vi "Util Convert to Base64url No Padding.vi"(11 "String (hex display)":string) -> (3 "Base64url String":string)   [LabVIEW 2020, in "Netatmo-WeatherStation.lvlib"]
doc: "This VI converts a string to its Base64 equivalent. Base64 strings are commonly used in Internet protocols such as HTTP, SMTP, etc."
uses:
  Netatmo-WeatherStation.lvlib
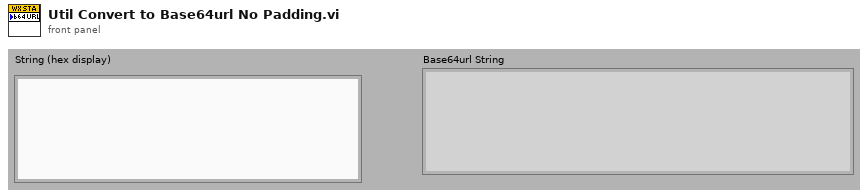
[diagram p1: front panel]
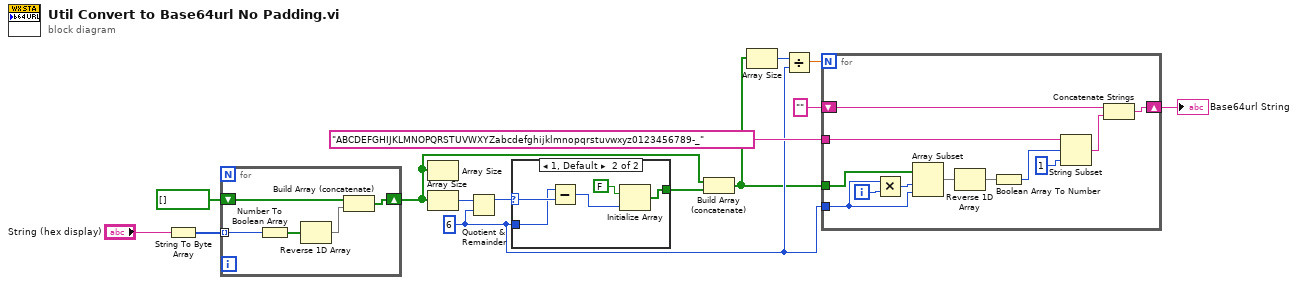
[diagram p0: block diagram]
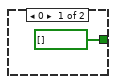
[diagram p2: hidden frame]
diagram:
  w4 = 6 ("y")
  n1 = String To Byte Array(string="String (hex display)") -> (unsigned byte array=w13:u8[])
  n2 = for {
    tunnel: w13 -> [w19] mode=indexing
    shift-right: [w16] -> w1
    shift-left: bool[] [] -> [w18]
    n3 = Number To Boolean Array(number=w19) -> (Boolean array=w17:bool[])
    n4 = Reverse 1D Array(array=w17) -> (reversed array=w15:bool[])
    n5 = Build Array (concatenate)(w18, w15) -> (w16:bool[])
  }
  n6 = Array Size(array=w1) -> ()  [unwired: 1 out]
  n7 = Array Size(array=w1) -> (size(s)=w7:i32)
  n8 = Quotient & Remainder(x=w7, y=w4) -> (x-y*floor(x/y)=w6:i32)  [unwired: 1 out]
  n9 = case shown="1, Default" w6 {
    selector: w6 -> [_ w24]
    tunnel: [bool[] [] w21] -> w5
    tunnel: w4 -> [_ w23]
    frame 0 {
    }
    frame 1, Default {
      n10 = Subtract(x=w23, y=w24) -> (x-y=w25:i32)
      n11 = Initialize Array(FALSE, w25) -> (w21:bool[])
    }
  }
  n12 = Build Array (concatenate)(w1, w5) -> (w3:bool[])
  n13 = Array Size(array=w3) -> (size(s)=w2:i32)
  n14 = Divide(x=w2, y=w4) -> (x/y=w8:dbl)
  n15 = for {
    N: w8 -> [_]
    tunnel: w3 -> [w36]
    tunnel: w4 -> [w34]
    tunnel: "ABCDEFGHIJKLMNOPQRSTUVWXYZabcdefghijklmnopqrstuvwxyz0123456789-_" -> [w33]
    shift-right: [w31] -> w9
    shift-left: "" -> [w30]
    i -> [w37]
    n16 = Multiply(x=w34, y=w37) -> (x*y=w35:i32)
    n17 = Array Subset(array=w36, index=w35, length=w34) -> (w26:bool[])
    n18 = Reverse 1D Array(array=w26) -> (reversed array=w27:bool[])
    n19 = Boolean Array To Number(Boolean array=w27) -> (number=w28:u32)
    n20 = String Subset(string=w33, offset (0)=w28, length (rest)=1 ("length (rest)")) -> (substring=w29:string)
    n21 = Concatenate Strings(w30, w29) -> (w31:string)
  }
  "Base64url String" <- w9
